vi "Do.vi"(8 "error in (no error)":errorcluster, 10 "Actor in":refnum<class "Actor.lvclass">, 11 "AcquireData":refnum<class "AcquireData.lvclass">) -> (0 "error out":errorcluster, 2 "Actor out":refnum<class "Actor.lvclass">)   [LabVIEW 2011, in "AcquireData.lvclass"]
doc: "(<B>Filename</B>: Actor Framework.lvlib:Message.lvclass:Do.vi)\n\nDefines what a message does when it is received by an actor. Generally, a message instructs an actor to invoke one of its methods.\n\nBy default, this method does nothing. A child class must override it to define behavior. Create a child class by using the Actor Framework Message Maker dialog box."
uses:
  AcquireData.lvclass
  <userlib>/_Frameworks/ActorFramework/Actor/Actor.lvclass
  Actors/DAQ/DAQ.lvclass
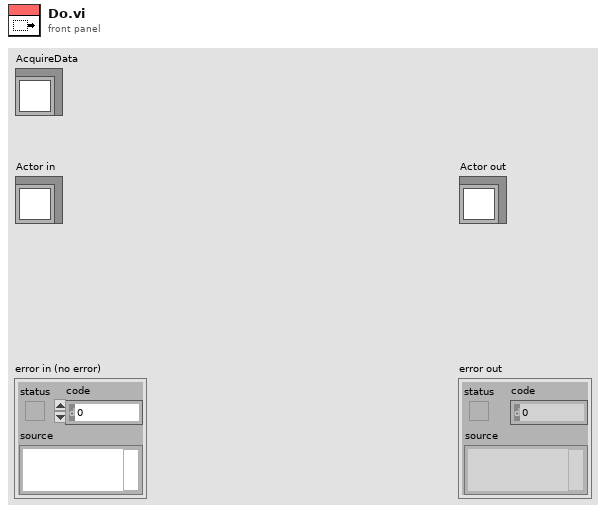
[diagram p1: front panel]
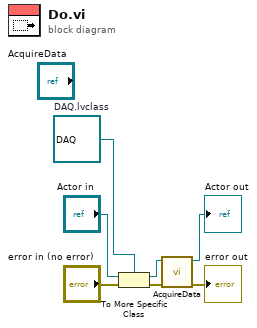
[diagram p0: block diagram]
diagram:
  w6 = refnum<class "DAQ.lvclass"> refnum  # DAQ.lvclass
  n1 = To More Specific Class(target class=w6, reference="Actor in", error in="error in (no error)") -> (specific class reference=w4:refnum<class "DAQ.lvclass">, error out=w3:errorcluster)
  n2 = call-dynamic "AcquireData.vi"("error in (no error)"=w3, "DAQ in"=w4) -> ("error out"=→"error out":errorcluster, "DAQ out"=→"Actor out":refnum<class "DAQ.lvclass">)  [unwired: 8 in]
